vi "Aerotech wait till acq stops.vi"(8 "error in (no error)":errorcluster) -> (0 "error out":errorcluster)   [LabVIEW 2020]
uses:
  Aerotech Acq FGV Function.ctl
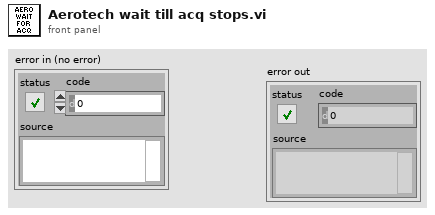
[diagram p1: front panel]
types:
  T1 = typedef "Aerotech Acq FGV Function.ctl" = enum16{"Clear", "Write", "Read"}
  T2 = typedef "Aerotech Acq FGV Control.ctl" = cluster{"Position":dbl[], "Power Status":bool[], "Move Active Status":bool[], "Busy Status":bool}
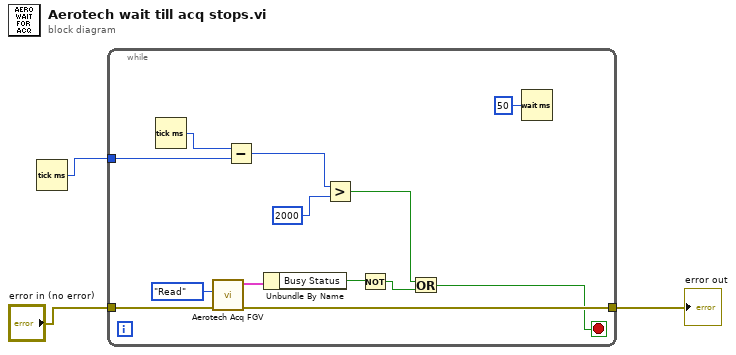
[diagram p0: block diagram]
diagram:
  n1 = Tick Count (ms)() -> (millisecond timer value=w1:u32)
  n2 = while {
    tunnel: "error in (no error)" -> [w16]
    tunnel: [w15] -> w2
    tunnel: w1 -> [w9]
    stop <- w5 stop-if-true
    n3 = Tick Count (ms)() -> (millisecond timer value=w10:u32)
    n4 = call "Aerotech Acq FGV.vi"("error in (no error)"=w16, "Function"=Aerotech_Acq_FGV_Function."Read") -> ("error out"=w15:errorcluster, "Aerotech Acq Data"=w13:T2)  [unwired: 8 in]
    n5 = Subtract(x=w10, y=w9) -> (x-y=w8:u32)
    n6 = Unbundle By Name(w13) -> ("Busy Status"=w12:bool)
    n7 = Greater?(x=w8, y=2000) -> (0:w6:bool)
    n8 = Not(x=w12) -> (.not. x?=w11:bool)
    n9 = Or(x=w6, y=w11) -> (x .or. y?=w5:bool)
    n10 = Wait (ms)(milliseconds to wait=u32 50) -> ()  [unwired: 1 out]
  }
  "error out" <- w2
